vi "Write spk.vi"(8 "error in (no error)":errorcluster, 10 "spk":bool, 11 "Speaker MSG in":refnum<class "Speaker MSG.lvclass">) -> (0 "error out":errorcluster, 3 "Speaker MSG out":refnum<class "Speaker MSG.lvclass">)   [LabVIEW 2014, in "Controller.lvlib" / "Speaker MSG.lvclass"]
uses:
  Speaker MSG.lvclass
  Speaker MSG.lvclass/Speaker MSG.ctl
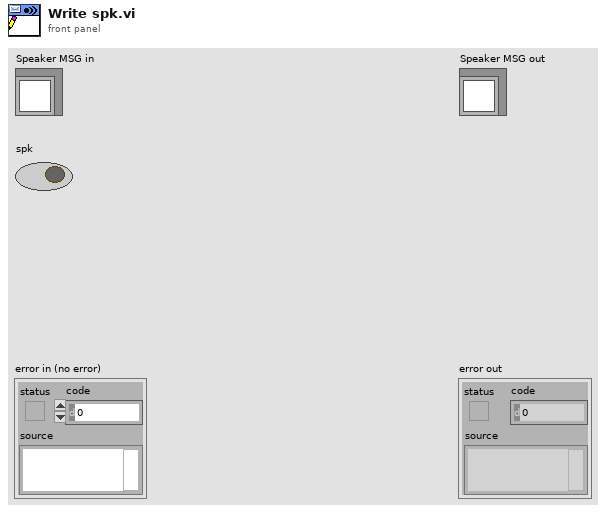
[diagram p1: front panel]
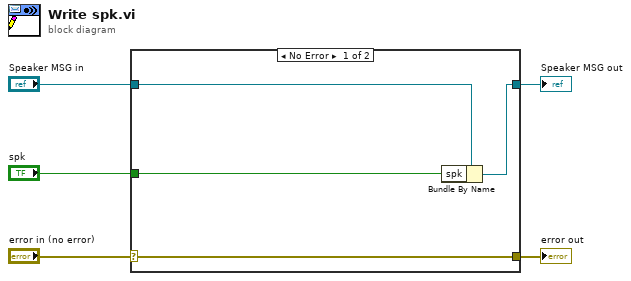
[diagram p0: block diagram]
diagram:
  n1 = case shown="No Error" "error in (no error)" {
    selector: "error in (no error)" -> [w9 w10]
    tunnel: [w9 w10] -> w4
    tunnel: [w7 w11] -> w2
    tunnel: "Speaker MSG in" -> [w8 w11]
    tunnel: "spk" -> [w6 _]
    frame No Error {
      n2 = Bundle By Name(cluster=w8, "spk"=w6) -> (w7:refnum<class "Speaker MSG.lvclass">)
    }
    frame Error {
    }
  }
  "error out" <- w4
  "Speaker MSG out" <- w2
